vi "write_params.vi"(8 "error in (no error)":errorcluster caption="entrée d'erreur (pas d'erreur)", 10 "params":T1={"n_neighbors"=5.0, "n_components"=2.0, "eigen_solver"="auto", "tol"=0.0, "max_iter"={"max_iter_type"="None", "max_iter_int"=0.0}, "path_method"="auto", "neighbors_algorithm"="auto", "n_jobs"=1.0, "metric"={"metric_type"="minkowski", "metric_function"=""}, "p"=2.0}, 11 "Isomap en entrée":refnum<class "Isomap.lvclass">) -> (0 "error out":errorcluster caption="sortie d'erreur", 3 "Isomap en sortie":refnum<class "Isomap.lvclass">)   [LabVIEW 2020, in "Isomap.lvclass"]
uses:
  Isomap.lvclass
  Controls/isomap_params.ctl
  Isomap.lvclass/Isomap.ctl
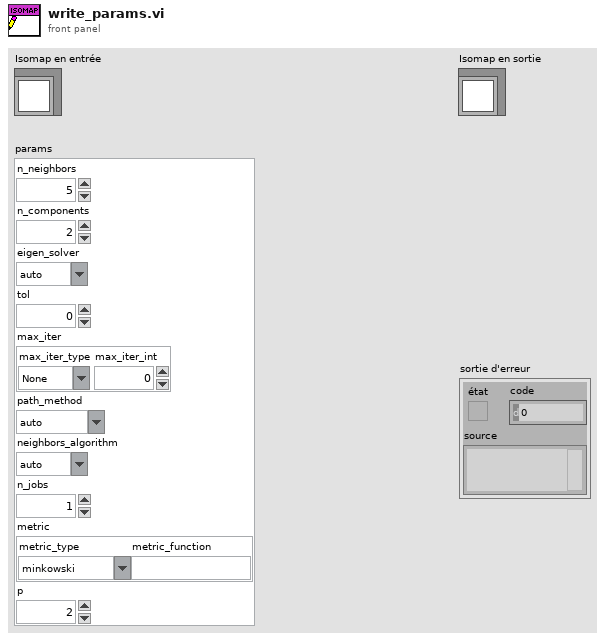
[diagram p1: front panel]
types:
  T1 = typedef "isomap_params.ctl" = cluster{"n_neighbors":dbl, "n_components":dbl, "eigen_solver":string, "tol":dbl, "max_iter":cluster{"max_iter_type":string, "max_iter_int":dbl}, "path_method":string, "neighbors_algorithm":string, "n_jobs":dbl, "metric":cluster{"metric_type":string, "metric_function":string}, "p":dbl}
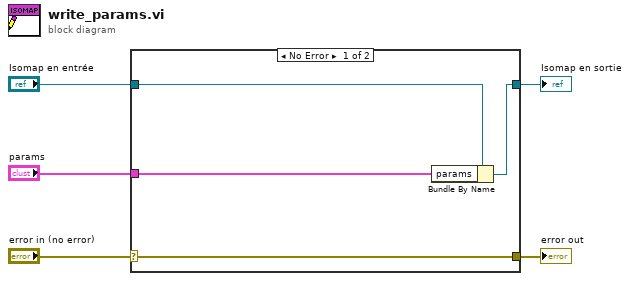
[diagram p0: block diagram]
diagram:
  n1 = case shown="No Error" "error in (no error)" {
    selector: "error in (no error)" -> [w9 w10]
    tunnel: [w9 w10] -> w4
    tunnel: [w7 w11] -> w2
    tunnel: "Isomap en entrée" -> [w8 w11]
    tunnel: "params" -> [w6 _]
    frame No Error {
      n2 = Bundle By Name(cluster=w8, "params"=w6) -> (w7:refnum<class "Isomap.lvclass">)
    }
    frame Error {
    }
  }
  "error out" <- w4
  "Isomap en sortie" <- w2
